vi "GraphLegend (SubVI).vi"(8 "error in (no error)":errorcluster, 11 "Graph":refnum<vi>[](array[refnum])) -> (0 "error out":errorcluster)   [LabVIEW 2017]
uses:
  Global_SNK3_HF.vi
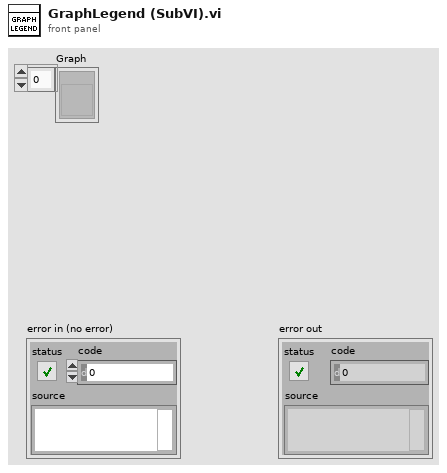
[diagram p1: front panel]
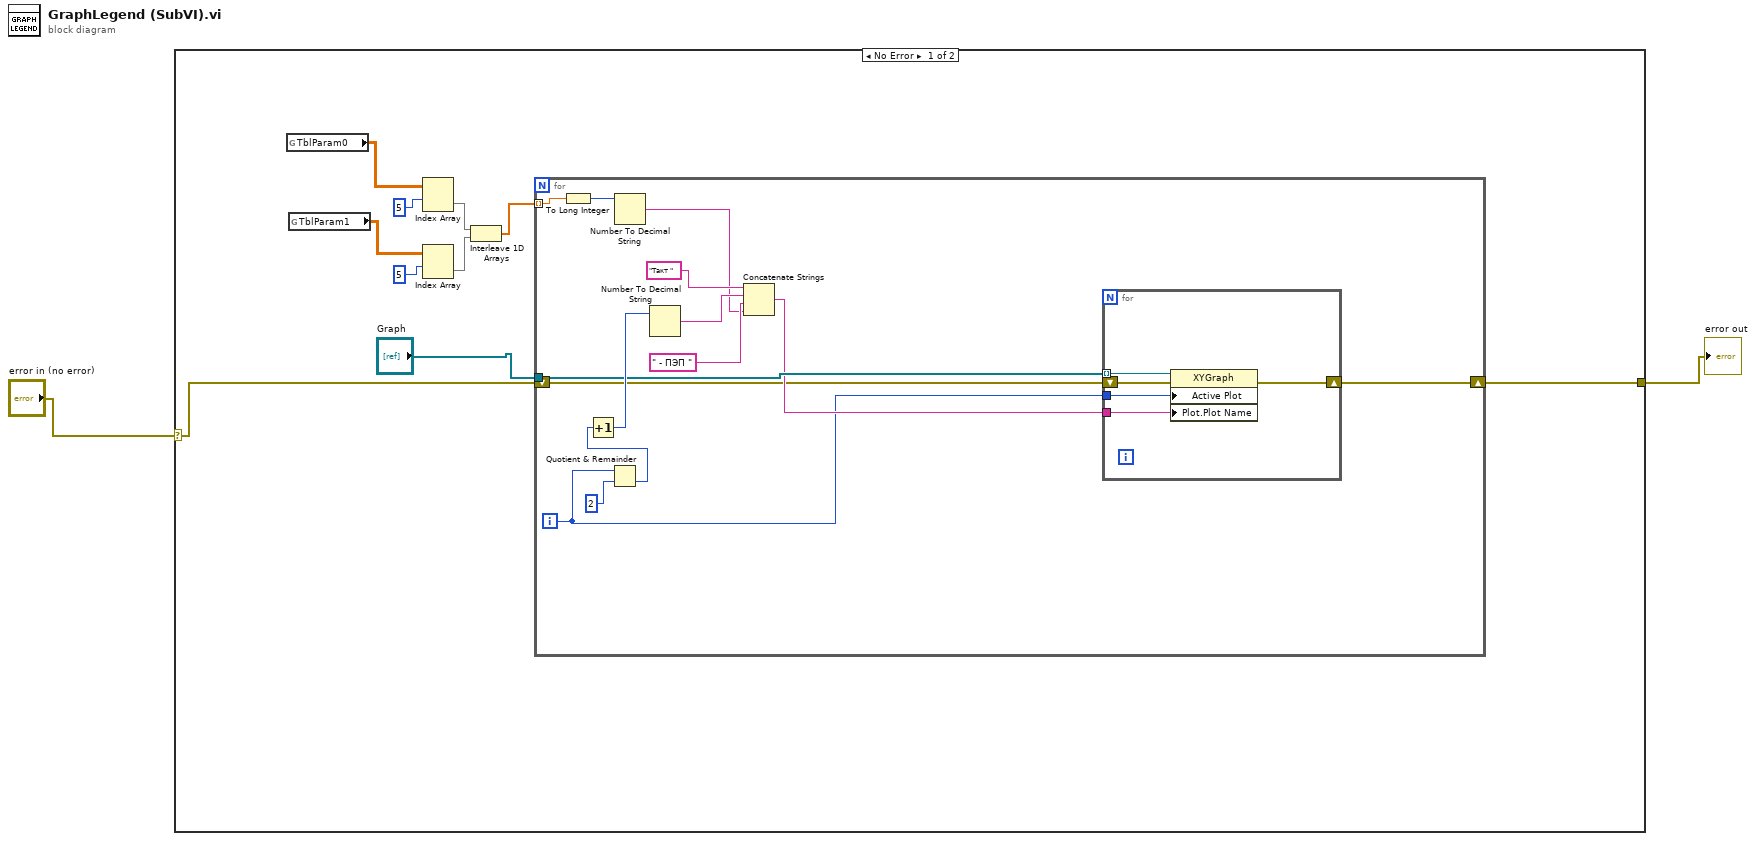
[diagram p0: block diagram]
diagram:
  n1 = case shown="No Error" "error in (no error)" {
    selector: "error in (no error)" -> [w3 w32]
    tunnel: [w4 w32] -> w1
    frame No Error {
      n2 = global read "Global_SNK3_HF.vi" "TblParam0"() -> (w8:sgl[][])
      n3 = global read "Global_SNK3_HF.vi" "TblParam1"() -> (w7:sgl[][])
      n4 = Index Array(array=w8, index (row)=5 ("disabled index (col)")) -> (element=w10:sgl[])  [unwired: 1 in]
      n5 = Index Array(array=w7, index (row)=5 ("disabled index (col)")) -> (element=w11:sgl[])  [unwired: 1 in]
      n6 = Interleave 1D Arrays(w10, w11) -> (w12:sgl[])
      n7 = for {
        tunnel: w12 -> [w22] mode=indexing
        tunnel: "Graph" -> [w17]
        shift-right: [w14] -> w4
        shift-left: w3 -> [w13]
        i -> [w15]
        n8 = To Long Integer(number=w22) -> (32bit integer=w21:i32)
        n9 = Quotient & Remainder(x=w15, y=2) -> (floor(x/y)=w18:i32)  [unwired: 1 out]
        n10 = Increment(x=w18) -> (x+1=w23:i32)
        n11 = Number To Decimal String(number=w21) -> (decimal integer string=w20:string)  [unwired: 1 in]
        n12 = Number To Decimal String(number=w23) -> (decimal integer string=w24:string)  [unwired: 1 in]
        n13 = Concatenate Strings("Такт " ("string"), w24, " - ПЭП " ("string"), w20) -> (w16:string)
        n14 = for {
          tunnel: w17 -> [w31] mode=indexing
          tunnel: w16 -> [w30]
          tunnel: w15 -> [w29]
          shift-right: [w28] -> w14
          shift-left: w13 -> [w27]
          n15 = property on="Property Node" class="XYGraph"(reference=w31, error in=w27, "Active Plot"=w29, "Plot.Plot Name"=w30) -> (error out=w28:errorcluster)  [unwired: 1 out]
        }
      }
    }
    frame Error {
    }
  }
  "error out" <- w1
